vi "Xenon Variable.vi"() -> ()   [LabVIEW 2010]
panel:
  out "Xenon Array":dbl[](array[numeric])
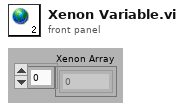
[diagram p1: front panel]
diagram:
